vi "geometricCupTesting.vi"() -> ()   [LabVIEW 2017]
panel:
  out "Y-Out":dbl
  out "X-Out":dbl
  out "CupPosition":T1(plugin-control)
  in  "File Path":path
  out "ImgToCrop":T1(plugin-control)
  out "Src Img":T1(plugin-control)
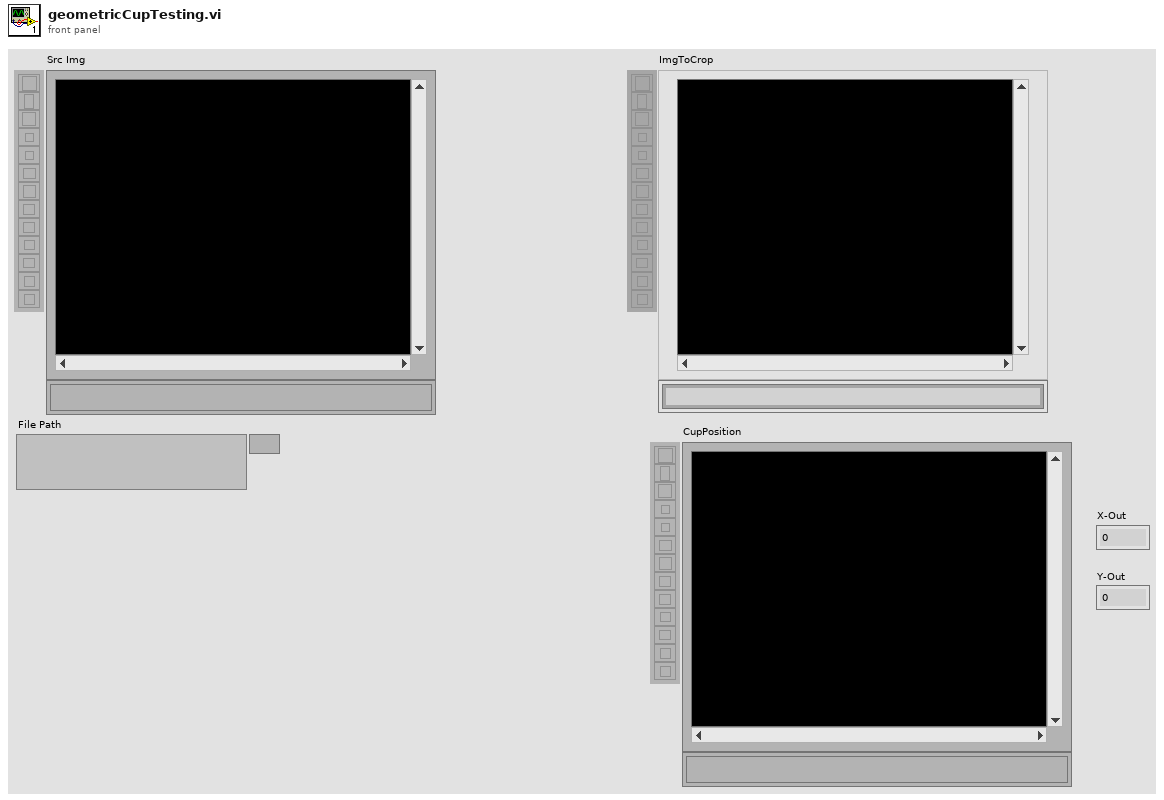
[diagram p1: front panel]
types:
  T1 = typedef "IMAQ Image.ctl" = refnum<image>
  T2 = typedef "Image Type" = u32
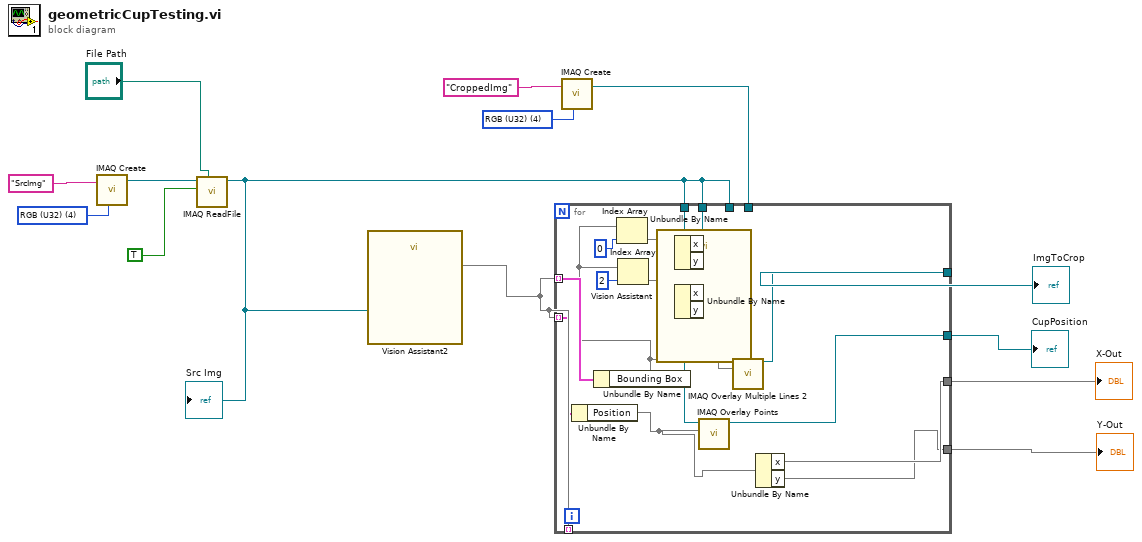
[diagram p0: block diagram]
diagram:
  w3 = T2 4 items=["Grayscale (U8)", "Grayscale (I16)", "Grayscale (SGL)", "Complex (CSG)", "RGB (U32)", "HSL (U32)", "RGB (U64)", "Grayscale (U16)"] ("Image Type")
  w13 = T2 4 items=["Grayscale (U8)", "Grayscale (I16)", "Grayscale (SGL)", "Complex (CSG)", "RGB (U32)", "HSL (U32)", "RGB (U64)", "Grayscale (U16)"] ("Image Type")
  n1 = call "IMAQ Create"("Image Name"="SrcImg", "Image Type"=w13) -> ("New Image"=w11:T1)  [unwired: 3 in, 1 out]
  n2 = call "IMAQ ReadFile"("File Path"="File Path", "Load Color Palette? (No)"=TRUE, "Image"=w11) -> ("Image Out"=w1:T1)  [unwired: 4 in, 4 out]
  "Src Img" <- w1
  n3 = call "Vision Assistant2"("Image In"=w1) -> (22:w5)  [unwired: 24 in, 2 out]
  n4 = call "IMAQ Create"("Image Name"="CroppedImg", "Image Type"=w3) -> ("New Image"=w2:T1)  [unwired: 3 in, 1 out]
  n5 = for {
    tunnel: [w22] -> w9
    tunnel: [w28] -> w8
    tunnel: [w27] -> w7
    tunnel: [w26] -> w6
    tunnel: w5 -> [_] mode=indexing
    tunnel: w1 -> [w25]
    tunnel: w1 -> [w24]
    tunnel: w5 -> [w23] mode=indexing
    tunnel: w5 -> [w21] mode=indexing
    tunnel: w2 -> [_]
    tunnel: w1 -> [_]
    n6 = Unbundle By Name(w23) -> ("Position"=w15)
    n7 = Unbundle By Name(w21) -> ("Bounding Box"=w18)
    n8 = Index Array(array=w18, index=0) -> (element=w19)
    n9 = Index Array(array=w18, index=2) -> (element=w16)
    n10 = Unbundle By Name(w19) -> ()  [unwired: 2 out]
    n11 = Unbundle By Name(w16) -> ()  [unwired: 2 out]
    n12 = call "IMAQ Overlay Points"("Point"=w15, "Image"=w24) -> ("Image Out"=w28:T1)  [unwired: 8 in, 1 out]
    n13 = call "IMAQ Overlay Multiple Lines 2"("Image"=w25, "Line End Points"=w18) -> ("Image Out"=w22:T1)  [unwired: 12 in, 1 out]
    n14 = Unbundle By Name(w15) -> ("x"=w27, "y"=w26)
  }
  "ImgToCrop" <- w9
  "CupPosition" <- w8
  "X-Out" <- w7
  "Y-Out" <- w6
  n15 = call "Vision Assistant"() -> ()  [unwired: 24 in, 4 out]
